vi "Create CArm.vi"(8 "error in (no error)":errorcluster, 11 "XRay CArm in":refnum<class "XRay CArm.lvclass">) -> (0 "error out":errorcluster, 3 "XRay CArm out":refnum<class "XRay CArm.lvclass">)   [LabVIEW 2026, in "XRay CArm.lvclass"]
uses:
  XRay CArm.lvclass
  XRay CArm.lvclass/XRay CArm.ctl
  <vilib>/picture/3D Picture Control/Object/Create Object (name).vi
  <vilib>/picture/3D Picture Control/Object/Add Object (no reference).vi
  <vilib>/picture/3D Picture Control/NI_3D Picture Control.lvlib
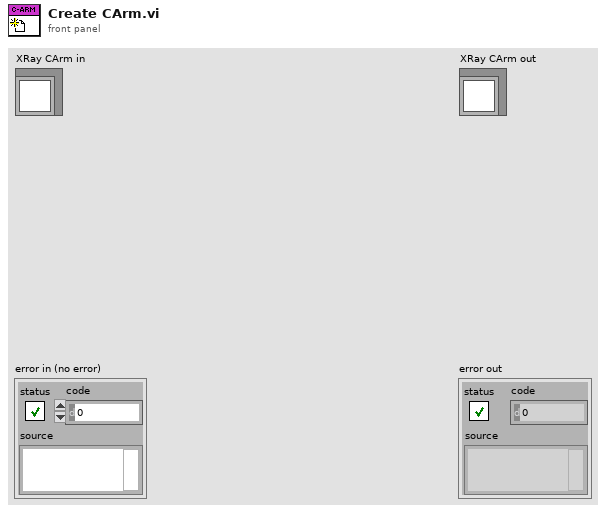
[diagram p1: front panel]
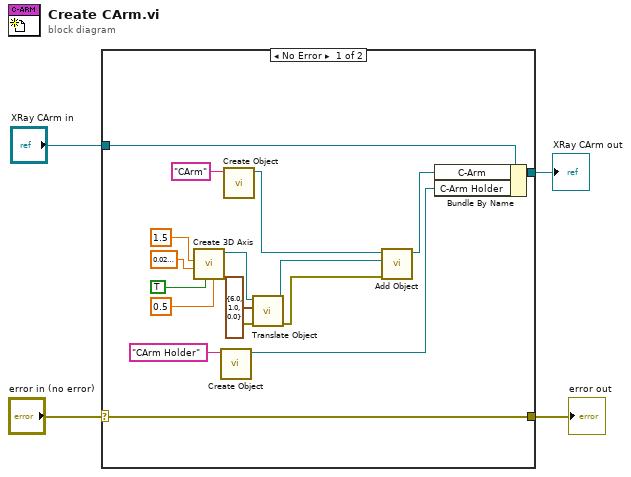
[diagram p0: block diagram]
diagram:
  n1 = case shown="No Error" "error in (no error)" {
    selector: "error in (no error)" -> [w18 w22]
    tunnel: [w18 w22] -> w3
    tunnel: [w20 w23] -> w1
    tunnel: "XRay CArm in" -> [w21 w23]
    frame No Error {
      n2 = call <vilib>:"Create 3D Axis.vi"("Character Size"=sgl 0.5, "Axis label?"=TRUE, "Radius"=sgl 0.03, "Length"=sgl 1.5 ("Height")) -> ("error out"=w9:errorcluster, "New Object Refnum"=w7:refnum<vi>)  [unwired: 6 in]
      n3 = call-poly <vilib>:"Create Object.vi"("Name"="CArm Holder") -> ("Scene:New Object"=w16:refnum<vi>)  [unwired: 9 in, 1 out]
      n4 = call-poly <vilib>:"Create Object.vi"("Name"="CArm") -> ("Scene:New Object"=w11:refnum<vi>)  [unwired: 9 in, 1 out]
      n5 = call <vilib>:"Translate Object.vi"("error in (no error)"=w9, "Translation"=cluster{"X":sgl, "Y":sgl, "Z":sgl} {"X"=6.0, "Y"=1.0, "Z"=0.0}, "Scene.Object In"=w7) -> ("error out"=w8:errorcluster, "Scene.Object Out"=w6:refnum<vi>)  [unwired: 7 in]
      n6 = call-poly <vilib>:"Add Object.vi"("error in (no error)"=w8, "New Object In"=w6, "Scene Object In"=w11) -> ("Scene Object Out"=w10:refnum<vi>)  [unwired: 7 in, 1 out]
      n7 = Bundle By Name(cluster=w21, "C-Arm"=w10, "C-Arm Holder"=w16) -> (w20:refnum<class "XRay CArm.lvclass">)
    }
    frame Error {
    }
  }
  "error out" <- w3
  "XRay CArm out" <- w1
